vi "getAdditionalDataXML.vi"(8 "error in (no error)":errorcluster, 11 "RfRamp in":refnum<class "RfRamp.lvclass">) -> (0 "error out":errorcluster, 2 "additionalDataXML":refnum<class "xmlNode.lvclass">, 3 "RfRamp out":refnum<class "RfRamp.lvclass">)   [LabVIEW 2009, in "Tools.lvlib" / "Scripting.lvlib" / "RfRamp.lvclass"]
uses:
  RfRamp.lvclass
  xmlNode/xmlNode.lvclass
  RfRamp.lvclass/RfRamp.ctl
  ScriptEvent.lvclass
  Rf Event/rf.lvclass
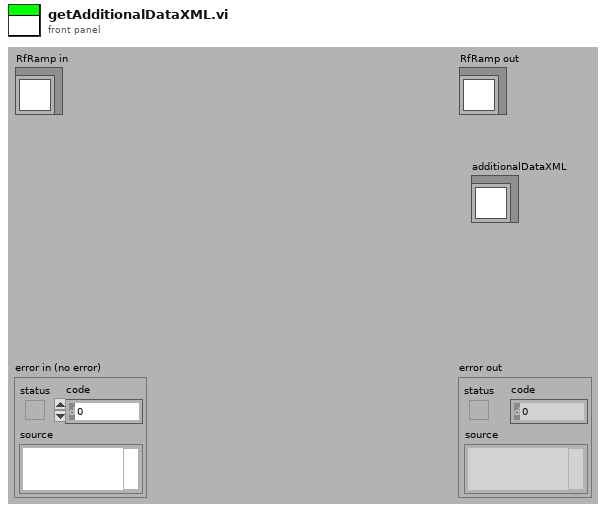
[diagram p1: front panel]
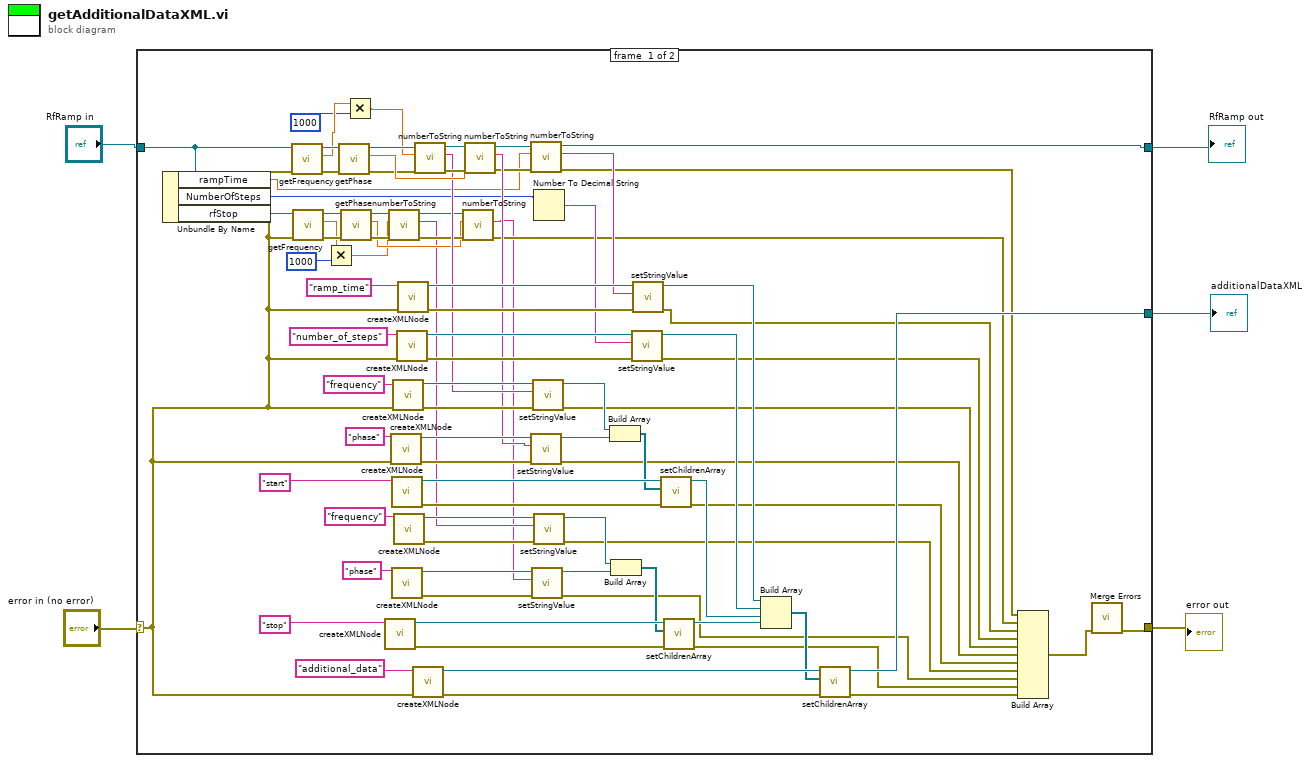
[diagram p0: block diagram]
diagram:
  n1 = case shown="No Error" "error in (no error)" {
    selector: "error in (no error)" -> [w69 w92]
    tunnel: [w16 w92] -> w3
    tunnel: [w14 w93] -> w1
    tunnel: "RfRamp in" -> [w77 w93]
    tunnel: [w84 _] -> w2
    frame #0 {
      n2 = Unbundle By Name(w77) -> ("rampTime"=w47:dbl, "NumberOfSteps"=w46:i32, "rfStop"=w76:refnum<class "rf.lvclass">)
      n3 = call "getFrequency.vi"("error in (no error)"=w69, "rf in"=w77) -> ("error out"=w62:errorcluster, "frequency"=w11:dbl, "rf out"=w63:refnum<class "RfRamp.lvclass">)  [unwired: 7 in]
      n4 = call "getFrequency.vi"("error in (no error)"=w69, "rf in"=w76) -> ("error out"=w55:errorcluster, "frequency"=w8:dbl, "rf out"=w56:refnum<class "rf.lvclass">)  [unwired: 7 in]
      n5 = Multiply(x=w8, y=1000) -> (x*y=w7:dbl)
      n6 = call "getPhase.vi"("error in (no error)"=w62, "rf in"=w63) -> ("error out"=w59:errorcluster, "phase"=w61:dbl, "rf out"=w60:refnum<class "RfRamp.lvclass">)  [unwired: 7 in]
      n7 = call "getPhase.vi"("error in (no error)"=w55, "rf in"=w56) -> ("error out"=w51:errorcluster, "phase"=w50:dbl, "rf out"=w52:refnum<class "rf.lvclass">)  [unwired: 7 in]
      n8 = Multiply(x=w11, y=1000) -> (x*y=w9:dbl)
      n9 = call "createXMLNode.vi"("name"="stop") -> ("error out"=w34:errorcluster, "xmlNode out"=w35:refnum<class "xmlNode.lvclass">)  [unwired: 9 in]
      n10 = call "numberToString.vi"("error in (no error)"=w51, "Numeric"=w7, "ScriptEvent in"=w52) -> ("error out"=w54:errorcluster, "String"=w13:string, "ScriptEvent out"=w53:refnum<class "rf.lvclass">)  [unwired: 6 in]
      n11 = call "createXMLNode.vi"("error in (no error)"=w69, "name"="phase") -> ("error out"=w81:errorcluster, "xmlNode out"=w82:refnum<class "xmlNode.lvclass">)  [unwired: 8 in]
      n12 = call "createXMLNode.vi"("name"="start") -> ("error out"=w65:errorcluster, "xmlNode out"=w66:refnum<class "xmlNode.lvclass">)  [unwired: 9 in]
      n13 = call "createXMLNode.vi"("name"="phase") -> ("error out"=w37:errorcluster, "xmlNode out"=w38:refnum<class "xmlNode.lvclass">)  [unwired: 9 in]
      n14 = call "createXMLNode.vi"("error in (no error)"=w69, "name"="frequency") -> ("error out"=w89:errorcluster, "xmlNode out"=w90:refnum<class "xmlNode.lvclass">)  [unwired: 8 in]
      n15 = call "createXMLNode.vi"("name"="frequency") -> ("error out"=w41:errorcluster, "xmlNode out"=w42:refnum<class "xmlNode.lvclass">)  [unwired: 9 in]
      n16 = call "createXMLNode.vi"("error in (no error)"=w69, "name"="number_of_steps") -> ("error out"=w71:errorcluster, "xmlNode out"=w72:refnum<class "xmlNode.lvclass">)  [unwired: 8 in]
      n17 = call "createXMLNode.vi"("error in (no error)"=w69, "name"="ramp_time") -> ("error out"=w74:errorcluster, "xmlNode out"=w75:refnum<class "xmlNode.lvclass">)  [unwired: 8 in]
      n18 = call "createXMLNode.vi"("error in (no error)"=w69, "name"="additional_data") -> ("error out"=w86:errorcluster, "xmlNode out"=w88:refnum<class "xmlNode.lvclass">)  [unwired: 8 in]
      n19 = call "numberToString.vi"("error in (no error)"=w59, "Numeric"=w9, "ScriptEvent in"=w60) -> ("error out"=w80:errorcluster, "String"=w58:string, "ScriptEvent out"=w79:refnum<class "RfRamp.lvclass">)  [unwired: 6 in]
      n20 = call "numberToString.vi"("error in (no error)"=w54, "Numeric"=w50, "ScriptEvent in"=w53) -> ("error out"=w18:errorcluster, "String"=w12:string)  [unwired: 6 in, 1 out]
      n21 = call "numberToString.vi"("error in (no error)"=w80, "Numeric"=w61, "ScriptEvent in"=w79) -> ("error out"=w48:errorcluster, "String"=w57:string, "ScriptEvent out"=w49:refnum<class "RfRamp.lvclass">)  [unwired: 6 in]
      n22 = call "numberToString.vi"("error in (no error)"=w48, "Numeric"=w47, "ScriptEvent in"=w49) -> ("error out"=w17:errorcluster, "String"=w44:string, "ScriptEvent out"=w14:refnum<class "RfRamp.lvclass">)  [unwired: 6 in]
      n23 = call-dynamic "setStringValue.vi"("error in (no error)"=w81, "stringValue"=w57, "xmlNode.lvclass in"=w82) -> ("error out"=w22:errorcluster, "xmlNode.lvclass out"=w78:refnum<class "xmlNode.lvclass">)  [unwired: 7 in]
      n24 = call-dynamic "setStringValue.vi"("error in (no error)"=w37, "stringValue"=w12, "xmlNode.lvclass in"=w38) -> ("error out"=w25:errorcluster, "xmlNode.lvclass out"=w36:refnum<class "xmlNode.lvclass">)  [unwired: 7 in]
      n25 = call-dynamic "setStringValue.vi"("error in (no error)"=w89, "stringValue"=w58, "xmlNode.lvclass in"=w90) -> ("error out"=w21:errorcluster, "xmlNode.lvclass out"=w85:refnum<class "xmlNode.lvclass">)  [unwired: 7 in]
      n26 = Number To Decimal String(number=w46) -> (decimal integer string=w45:string)  [unwired: 1 in]
      n27 = call-dynamic "setStringValue.vi"("error in (no error)"=w41, "stringValue"=w13, "xmlNode.lvclass in"=w42) -> ("error out"=w24:errorcluster, "xmlNode.lvclass out"=w40:refnum<class "xmlNode.lvclass">)  [unwired: 7 in]
      n28 = Build Array(w85, w78) -> (w64:refnum<class "xmlNode.lvclass">[])
      n29 = Build Array(w40, w36) -> (w33:refnum<class "xmlNode.lvclass">[])
      n30 = call-dynamic "setStringValue.vi"("error in (no error)"=w71, "stringValue"=w45, "xmlNode.lvclass in"=w72) -> ("error out"=w20:errorcluster, "xmlNode.lvclass out"=w31:refnum<class "xmlNode.lvclass">)  [unwired: 7 in]
      n31 = call-dynamic "setStringValue.vi"("error in (no error)"=w74, "stringValue"=w44, "xmlNode.lvclass in"=w75) -> ("error out"=w19:errorcluster, "xmlNode.lvclass out"=w32:refnum<class "xmlNode.lvclass">)  [unwired: 7 in]
      n32 = call-dynamic "setChildrenArray.vi"("error in (no error)"=w65, "Children"=w64, "xmlNode.lvclass in"=w66) -> ("error out"=w23:errorcluster, "xmlNode.lvclass out"=w30:refnum<class "xmlNode.lvclass">)  [unwired: 7 in]
      n33 = call-dynamic "setChildrenArray.vi"("error in (no error)"=w34, "Children"=w33, "xmlNode.lvclass in"=w35) -> ("error out"=w26:errorcluster, "xmlNode.lvclass out"=w29:refnum<class "xmlNode.lvclass">)  [unwired: 7 in]
      n34 = Build Array(w32, w31, w30, w29) -> (w28:refnum<class "xmlNode.lvclass">[])
      n35 = call-dynamic "setChildrenArray.vi"("error in (no error)"=w86, "Children"=w28, "xmlNode.lvclass in"=w88) -> ("error out"=w27:errorcluster, "xmlNode.lvclass out"=w84:refnum<class "xmlNode.lvclass">)  [unwired: 7 in]
      n36 = Build Array(w17, w18, w19, w20, w21, w22, w23, w24, w25, w26, w27) -> (w15:errorcluster[])
      n37 = call <vilib>:"Merge Errors.vi"("error array in"=w15) -> ("error out"=w16:errorcluster)  [unwired: 6 in]
    }
    frame #1 {
    }
  }
  "error out" <- w3
  "RfRamp out" <- w1
  "additionalDataXML" <- w2
